vi "BUILD_read full file.vi"(8 "error in":errorcluster, 11 "vip file":path) -> (0 "error out":errorcluster, 3 "data":string)   [LabVIEW 2010]
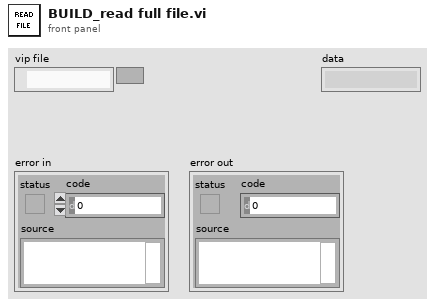
[diagram p1: front panel]
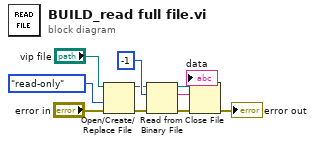
[diagram p0: block diagram]
diagram:
  n1 = Open/Create/Replace File(file path (use dialog)="vip file", error in="error in", access (0:read/write)=enum16{"read/write", "read-only", "write-only"}."read-only") -> (refnum out=w5:refnum<file>, error out=w6:errorcluster)  [unwired: 3 in, 1 out]
  n2 = Read from Binary File(8:w6, 10:-1 ("count (1)"), 11:w5) -> (0:w9:errorcluster, 2:→"data":string, 3:w8:refnum<file>)  [unwired: 3 in, 1 out]
  n3 = Close File(refnum=w8, error in=w9) -> (error out=→"error out":errorcluster)  [unwired: 1 out]
